vi "Autofocus.vi"(8 "error in (no error)":errorcluster, 9 "Range":dbl=0.2, 10 "Crop Factor":dbl, 11 "Gantry in":refnum<class "Gantry.lvclass">) -> (0 "error out":errorcluster, 2 "Focus Point":refnum<class "Vec3d.lvclass">, 3 "Gantry out":refnum<class "Gantry.lvclass">)   [LabVIEW 2024, in "Gantry.lvclass"]
uses:
  Gantry.lvclass
  Vec3d Class/Vec3d.lvclass
  FlexWorktable/FlexWorktable.lvclass
  Vision/Vision.lvlib
panel:
  out "Live Preview":T1(plugin-control)
  out "result":string="Fit Result: -"
  out "progress":string="-"
  out "XY Graph":cluster{"X":dbl, "Y":dbl}[](graph)
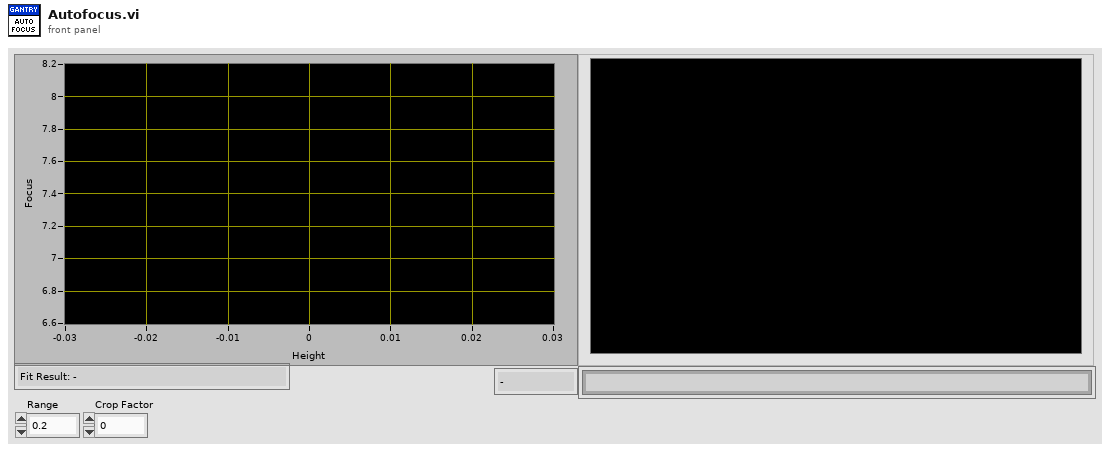
[diagram p1: front panel]
types:
  T1 = typedef "IMAQ Image.ctl" = refnum<image>
  T2 = typedef "Physical Image.ctl" = cluster{"Image Position":refnum<class "Vec3d.lvclass">, "Image Reference":T1, "Field of View":cluster{"x(mm)":dbl, "y(mm)":dbl}}
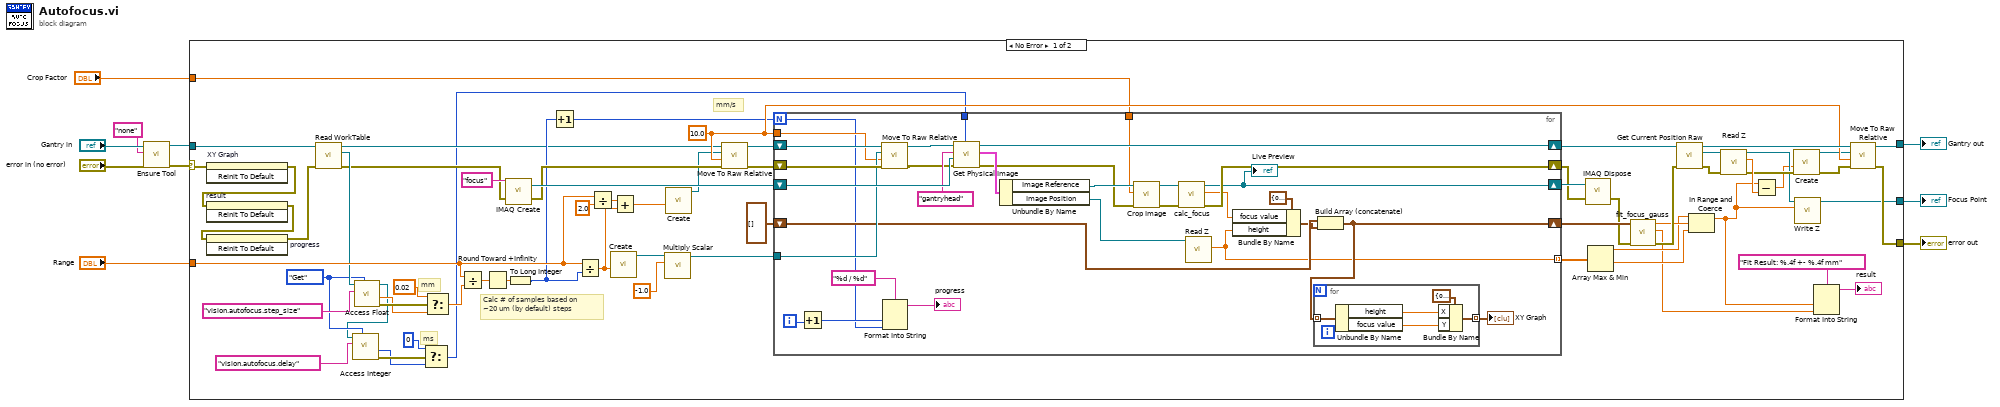
[diagram p0: block diagram]
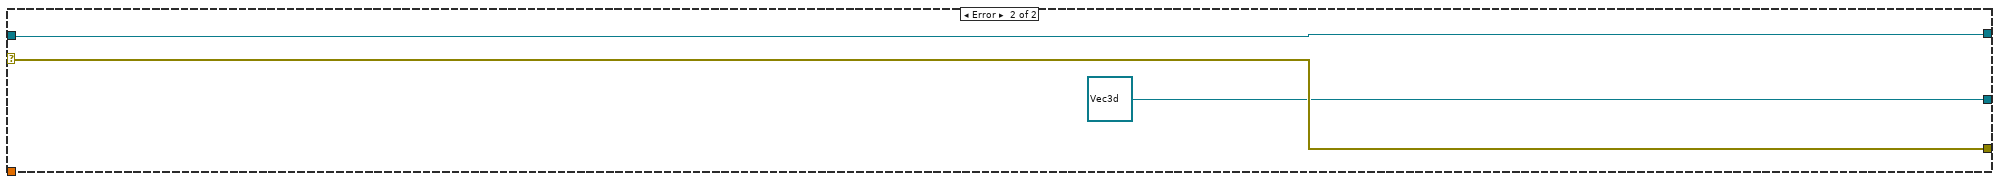
[diagram p2: hidden frame]
diagram:
  n1 = call "Ensure Tool.vi"("error in (no error)"="error in (no error)", "Tool Name"="none", "Gantry in"="Gantry in") -> ("error out"=w5:errorcluster, "Gantry out"=w4:refnum<class "Gantry.lvclass">)  [unwired: 7 in]
  n2 = case shown="No Error" w5 {
    selector: w5 -> [w46 w115]
    tunnel: w4 -> [w36 w116]
    tunnel: [w53 w115] -> w8
    tunnel: [w54 w116] -> w9
    tunnel: "Range" -> [w77 _]
    tunnel: [w16 refnum<class "Vec3d.lvclass"> refnum ("Vec3d Class out")] -> w2
    tunnel: "Crop Factor" -> [w11 _]
    frame No Error {
      w21 = enum16{"Get", "Set"}."Get" ("Get/Set")
      w55 = 10.0 ("Speed(mm/s)")
      # "mm"
      # "ms"
      # "mm/s"
      # "Calc # of samples based on\n~20 um (by default) steps"
      n3 = invoke on="XY Graph" class="XYGraph (strict)" method="Reinit To Default"(error in=w46) -> (error out=w38:errorcluster)  [unwired: 2 in, 2 out]
      n4 = invoke on="result" class="Str" method="Reinit To Default"(error in=w38) -> (error out=w37:errorcluster)  [unwired: 2 in, 2 out]
      n5 = invoke on="progress" class="Str" method="Reinit To Default"(error in=w37) -> (error out=w35:errorcluster)  [unwired: 2 in, 2 out]
      n6 = call-dynamic "Read WorkTable.vi"("error in"=w35, "Gantry Class in"=w36) -> ("error out"=w32:errorcluster, "Worktable"=w33:refnum<class "FlexWorktable.lvclass">, "Gantry Class out"=w34:refnum<class "Gantry.lvclass">)  [unwired: 7 in]
      n7 = call-dynamic "Access Float.vi"("Get/Set"=w21, "Key"="vision.autofocus.step_size", "FlexWorktable in"=w33) -> ("error out"=w30:errorcluster, "Value out"=w28:dbl, "FlexWorktable out"=w20:refnum<class "FlexWorktable.lvclass">)  [unwired: 6 in]
      n8 = call-dynamic "Access Integer.vi"("Get/Set"=w21, "Key"="vision.autofocus.delay", "FlexWorktable in"=w20) -> ("error out"=w25:errorcluster, "Value out"=w23:i32)  [unwired: 6 in, 1 out]
      n9 = Select(t=0 ("y"), s=w25, f=w23) -> (s? t:f=w22:i32)
      n10 = Select(t=0.02 ("y"), s=w30, f=w28) -> (s? t:f=w27:dbl)
      n11 = Divide(x=w77, y=w27) -> (x/y=w72:dbl)
      n12 = Round Toward +Infinity(x=w72) -> (ceil(x): smallest int >= x=w71:dbl)
      n13 = call "IMAQ Create"("Image Name"="focus", "error in (no error)"=w32) -> ("New Image"=w75:T1, "error out"=w68:errorcluster)  [unwired: 3 in]
      n14 = To Long Integer(number=w71) -> (32bit integer=w47:i32)
      n15 = Increment(x=w47) -> (x+1=w48:i32)
      n16 = Divide(x=w77, y=w47) -> (x/y=w51:dbl)
      n17 = Divide(x=w77, y=2.0) -> (x/y=w52:dbl)
      n18 = call "Create.vi"("Z"=w51) -> ("Vec3d Class out"=w64:refnum<class "Vec3d.lvclass">)  [unwired: 9 in, 1 out]
      n19 = Add(x=w52, y=w51) -> (x+y=w49:dbl)
      n20 = call-dynamic "Multiply Scalar.vi"("Scale"=-1.0, "Vec3d in"=w64) -> ("Vec3d out"=w62:refnum<class "Vec3d.lvclass">)  [unwired: 8 in, 1 out]
      n21 = call "Create.vi"("Z"=w49) -> ("Vec3d Class out"=w50:refnum<class "Vec3d.lvclass">)  [unwired: 9 in, 1 out]
      n22 = call-dynamic "Move To Raw Relative.vi"("error in"=w68, "Speed(mm/s)"=w55, "Delta"=w50, "Gantry in"=w34) -> ("error out"=w66:errorcluster, "Gantry out"=w65:refnum<class "Gantry.lvclass">)  [unwired: 6 in]
      n23 = for {
        N: w48 -> [w87]
        shift-right: [w108] -> w61
        shift-left: w65 -> [w98]
        shift-right: [w107] -> w70
        shift-left: w66 -> [w100]
        shift-right: [w78] -> w74
        shift-left: w75 -> [w106]
        tunnel: w62 -> [w99]
        tunnel: w55 -> [w97]
        shift-right: [w91] -> w73
        shift-left: cluster{"focus value":dbl, "height":dbl}[] [] -> [w93]
        tunnel: [w85] -> w45 mode=indexing
        tunnel: w22 -> [w84]
        tunnel: w11 -> [w80]
        i -> [w89]
        n24 = Increment(x=w89) -> (x+1=w88:i32)
        n25 = call-dynamic "Move To Raw Relative.vi"("error in"=w100, "Speed(mm/s)"=w97, "Delta"=w99, "Gantry in"=w98) -> ("error out"=w95:errorcluster, "Gantry out"=w96:refnum<class "Gantry.lvclass">)  [unwired: 6 in]
        n26 = Format Into String(format string="%d / %d", w88, w87) -> (resulting string=→"progress":string)  [unwired: 2 in, 1 out]
        n27 = call-dynamic "Get Physical Image.vi"("Delay(milliseconds)"=w84, "error in"=w95, "Image In"=w106, "Camera Name"="gantryhead", "Gantry in"=w96) -> ("error out"=w82:errorcluster, "Physical Image"=w103:T2, "Gantry out"=w108:refnum<class "Gantry.lvclass">)  [unwired: 4 in]
        n28 = Unbundle By Name(w103) -> ("Image Reference"=w83:T1, "Image Position"=w102:refnum<class "Vec3d.lvclass">)
        n29 = call "Crop Image.vi"("error in (no error)"=w82, "Crop Factor"=w80, "Source Image"=w83) -> ("error out"=w81:errorcluster, "Cropped Image"=w79:T1)  [unwired: 7 in]
        n30 = call "calc_focus.vi"("error in"=w81, "Image"=w79) -> ("error out"=w107:errorcluster, "focus"=w104:sgl, "Image out"=w78:T1)  [unwired: 7 in]
        "Live Preview" <- w78
        n31 = call-dynamic "Read Z.vi"("Vec3d Class in"=w102) -> ("Z"=w85:dbl)  [unwired: 8 in, 2 out]
        n32 = Bundle By Name(cluster=cluster{"focus value":dbl, "height":dbl} {"focus value"=0.0, "height"=0.0} ("Focus Measurement"), "focus value"=w104, "height"=w85) -> (w92:cluster{"focus value":dbl, "height":dbl})
        n33 = Build Array (concatenate)(w93, w92) -> (w91:cluster{"focus value":dbl, "height":dbl}[])
        n34 = for {
          tunnel: w91 -> [w113] mode=indexing
          tunnel: [w110] -> w94 mode=indexing
          n35 = Unbundle By Name(w113) -> ("height"=w109:dbl, "focus value"=w111:dbl)
          n36 = Bundle By Name(cluster=cluster{"X":dbl, "Y":dbl} {"X"=0.0, "Y"=0.0}, "X"=w109, "Y"=w111) -> (w110:cluster{"X":dbl, "Y":dbl})
        }
        "XY Graph" <- w94
      }
      n37 = call "IMAQ Dispose"("Image"=w74, "error in (no error)"=w70) -> ("error out"=w69:errorcluster)  [unwired: 4 in]
      n38 = Array Max & Min(array=w45) -> (max value=w43:dbl, min value=w42:dbl)  [unwired: 2 out]
      n39 = call "fit_focus_gauss.vi"("error in"=w69, "Focus Measurements"=w73) -> ("error out"=w57:errorcluster, "error"=w39:dbl, "focus height"=w44:dbl)  [unwired: 7 in]
      n40 = call-dynamic "Get Current Position Raw.vi"("error in"=w57, "Gantry in"=w61) -> ("error out"=w56:errorcluster, "Vec3d Class out"=w60:refnum<class "Vec3d.lvclass">, "Gantry out"=w58:refnum<class "Gantry.lvclass">)  [unwired: 7 in]
      n41 = In Range and Coerce(upper limit=w43, x=w44, lower limit=w42) -> (coerced(x)=w13:dbl)  [unwired: 1 out]
      n42 = call-dynamic "Read Z.vi"("error in (no error)"=w56, "Vec3d Class in"=w60) -> ("error out"=w19:errorcluster, "Z"=w59:dbl, "Vec3d Class out"=w15:refnum<class "Vec3d.lvclass">)  [unwired: 7 in]
      n43 = Subtract(x=w13, y=w59) -> (x-y=w14:dbl)
      n44 = call "Create.vi"("error in"=w19, "Z"=w14) -> ("error out"=w17:errorcluster, "Vec3d Class out"=w18:refnum<class "Vec3d.lvclass">)  [unwired: 8 in]
      n45 = call-dynamic "Write Z.vi"("Z"=w13, "Vec3d Class in"=w15) -> ("Vec3d Class out"=w16:refnum<class "Vec3d.lvclass">)  [unwired: 8 in, 1 out]
      n46 = Format Into String(format string="Fit Result: %.4f +- %.4f mm", w13, w39) -> (resulting string=→"result":string)  [unwired: 2 in, 1 out]
      n47 = call-dynamic "Move To Raw Relative.vi"("error in"=w17, "Speed(mm/s)"=w55, "Delta"=w18, "Gantry in"=w58) -> ("error out"=w53:errorcluster, "Gantry out"=w54:refnum<class "Gantry.lvclass">)  [unwired: 6 in]
    }
    frame Error {
    }
  }
  "error out" <- w8
  "Gantry out" <- w9
  "Focus Point" <- w2
